vi "Process File.vi"(8 "error in (no error)":errorcluster, 10 "Result in":refnum<class "Acquired Result.lvclass">, 11 "Strain Logger in":refnum<class "Strain Logger.lvclass">) -> (0 "error out":errorcluster, 2 "Result out":refnum<class "Acquired Result.lvclass">, 3 "Strain Logger out":refnum<class "Strain Logger.lvclass">)   [LabVIEW 2024, in "Strain Logger.lvclass"]
uses:
  Strain Logger.lvclass
  NHMFL_Core/Libraries/Instruments/Results/Acquired Result/Acquired Result.lvclass
  Strain Logger.lvclass/Strain Logger.ctl
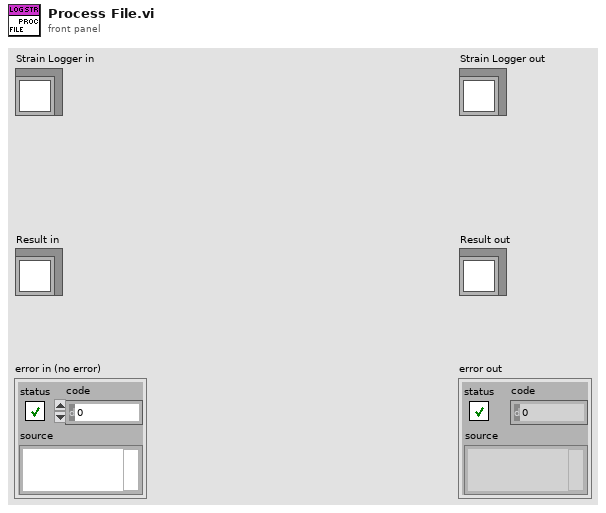
[diagram p1: front panel]
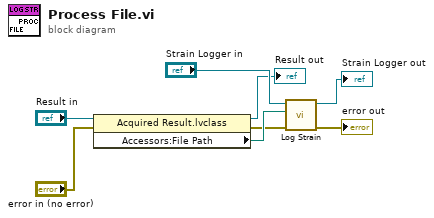
[diagram p0: block diagram]
diagram:
  n1 = property class="Acquired Result.lvclass"(reference="Result in", error in="error in (no error)") -> (reference out=→"Result out":refnum<class "Acquired Result.lvclass">, error out=w3:errorcluster, "Accessors:File Path"=w4:path)
  n2 = call-dynamic "Log Strain.vi"("error in (no error)"=w3, "Input file"=w4, "Strain Logger in"="Strain Logger in") -> ("error out"=→"error out":errorcluster, "Strain Logger out"=→"Strain Logger out":refnum<class "Strain Logger.lvclass">)  [unwired: 7 in]
